vi "main(Test DQMH modules).vi"() -> ()   [LabVIEW 2018, in "Application.lvlib"] (continued)
          }
        }
        n5217 = for {
          tunnel: w11392 -> [w11487] mode=indexing
          tunnel: w11400 -> [w11488]
          tunnel: [w11484] -> w11402 mode=indexing
          n5218 = Unbundle By Name(w11487) -> ("command"=w11486:string, "data"=w11485:variant)
          n5219 = call "App enquece.vi"("command data"=w11485, "command"=w11486, "queue in"=w11488) -> ("error out"=w11484:errorcluster)  [unwired: 7 in, 1 out]
        }
        n5220 = Merge Errors(w11403, w11402) -> (w11401:errorcluster)
      }
      frame "Test DRV 17A" {
        w11492 = 17 ("DUT index(0-59)")
        n5221 = disable-structure shown="LOGGING==TRUE" {
          disable-tunnel: w11497 -> [w11580 _]
          frame condition #0 (active) {
            n5222 = Empty String/Path?(string/path=w11580) -> (empty?=w11582:bool)
            n5223 = Select(t="Quece timeout", s=w11582, f=w11580) -> (s? t:f=w11579:string)
            n5224 = call "string log (SubVI).vi"("state Name"=w11579) -> ()  [unwired: 9 in, 2 out]
          }
          frame condition #1 {
          }
        }
        n5225 = Flush Queue(queue=w11498) -> (queue out=w11499:refnum<queue>)  [unwired: 1 in, 2 out]
        n5226 = Decrement(x=w11492) -> (x-1=w11496:i32)
        n5227 = Index Array(array=w11493, index=w11496) -> (element=w11494:refnum<vi>)
        n5228 = call "FGV DRV stand.vi"() -> ("Sub-Test.DCV"=w11489:bool)  [unwired: 10 in, 1 out]
        n5229 = call "FGV Driver Data.vi"("DUT index(1-60)"=w11492) -> ("DUT SC"=w11490:bool)  [unwired: 7 in, 3 out]
        n5230 = property class="ColBox"(reference=w11494, "Value"=u32 10000536 ("DRV 1")) -> ()  [unwired: 1 in, 2 out]
        n5231 = case shown="False" w11490 {
          tunnel: w11492 -> [w11510 _]
          tunnel: [w11509 w11575] -> w11491
          tunnel: w11489 -> [w11508 _]
          frame False {
            n5232 = case shown="True" w11508 {
              tunnel: w11510 -> [w11517 w11547]
              tunnel: [w11528 w11546] -> w11509
              frame False {
                w11514 = T9 {"command"="", "data"=variant} ("element")
                w11527 = T9 {"command"="", "data"=variant} ("element")
                n5233 = To Variant(anything=T3."mux10_1_channel3" ("mux10_1(x6)_encode")) -> (Variant=w11525:variant)
                n5234 = To Variant(anything=T4."demux1_10_channel3" ("demux1_10(x6)_encode")) -> (Variant=w11521:variant)
                n5235 = To Variant(anything=bool[] [FALSE, FALSE, FALSE, FALSE, TRUE, FALSE]) -> (Variant=w11536:variant)
                n5236 = Bundle By Name(cluster=w11527, "command"="MEAS.AllRelaysOFF") -> (w11535:T9)
                n5237 = Bundle By Name(cluster=w11527, "command"="MEAS.mux10-1", "data"=w11525) -> (w11518:T9)
                n5238 = Bundle By Name(cluster=w11527, "command"="MEAS.demux1-10", "data"=w11521) -> (w11519:T9)
                n5239 = Bundle By Name(cluster=w11527, "command"="MEAS.eMIC", "data"=w11536) -> (w11520:T9)
                n5240 = Build Array(w11535, w11518, w11519, w11520) -> (w11513:T9[])
                n5241 = To Variant(anything=w11517) -> (Variant=w11516:variant)
                n5242 = To Variant(anything=w11517) -> (Variant=w11515:variant)
                n5243 = Bundle By Name(cluster=w11514, "command"="MEAS.requestAC", "data"=w11516) -> (w11533:T9)
                n5244 = Bundle By Name(cluster=w11514, "command"="Apps.WaitForEvent", "data"=w11515) -> (w11529:T9)
                n5245 = Bundle By Name(cluster=w11514, "command"="Apps.UI Update 1") -> (w11530:T9)
                n5246 = Bundle By Name(cluster=w11514, "command"="WaitFor") -> (w11512:T9)
                n5247 = Build Array (concatenate)(w11513, w11512, w11533, w11529, w11530) -> (w11528:T9[])
              }
              frame True {
                w11543 = T9 {"command"="", "data"=variant} ("element")
                w11565 = T9 {"command"="", "data"=variant} ("element")
                n5248 = To Variant(anything=T3."mux10_1_channel3" ("mux10_1(x6)_encode")) -> (Variant=w11572:variant)
                n5249 = To Variant(anything=T2."mux6_1_channel5_3" ("mux6_1(3wires)_encode")) -> (Variant=w11570:variant)
                n5250 = To Variant(anything=T4."demux1_10_channel3" ("demux1_10(x6)_encode")) -> (Variant=w11566:variant)
                n5251 = To Variant(anything=bool[] [FALSE, FALSE, FALSE, FALSE, TRUE, FALSE]) -> (Variant=w11562:variant)
                n5252 = Bundle By Name(cluster=w11565, "command"="MEAS.AllRelaysOFF") -> (w11561:T9)
                n5253 = Bundle By Name(cluster=w11565, "command"="MEAS.mux10-1", "data"=w11572) -> (w11560:T9)
                n5254 = Bundle By Name(cluster=w11565, "command"="MEAS.mux6_1", "data"=w11570) -> (w11559:T9)
                n5255 = Bundle By Name(cluster=w11565, "command"="MEAS.demux1-10", "data"=w11566) -> (w11558:T9)
                n5256 = Bundle By Name(cluster=w11565, "command"="MEAS.eMIC", "data"=w11562) -> (w11557:T9)
                n5257 = Build Array(w11561, w11560, w11559, w11558, w11557) -> (w11542:T9[])
                n5258 = To Variant(anything=w11547) -> (Variant=w11545:variant)
                n5259 = To Variant(anything=w11547) -> (Variant=w11544:variant)
                n5260 = Bundle By Name(cluster=w11543, "command"="WaitFor") -> (w11541:T9)
                n5261 = Bundle By Name(cluster=w11543, "command"="MEAS.DMM dual read") -> (w11554:T9)
                n5262 = Bundle By Name(cluster=w11543, "command"="MEAS.requestAC", "data"=w11545) -> (w11553:T9)
                n5263 = Bundle By Name(cluster=w11543, "command"="Apps.WaitForEvent", "data"=w11544) -> (w11548:T9)
                n5264 = Bundle By Name(cluster=w11543, "command"="Apps.UI Update 1") -> (w11549:T9)
                n5265 = Build Array (concatenate)(w11542, w11541, w11554, w11553, w11548, w11549) -> (w11546:T9[])
              }
            }
          }
          frame True {
            n5266 = Bundle By Name(cluster=T9 {"command"="", "data"=variant} ("element"), "command"="Apps.UI Update 1") -> (w11576:T9)
            n5267 = Build Array(w11576) -> (w11575:T9[])
          }
        }
        n5268 = for {
          tunnel: w11491 -> [w11586] mode=indexing
          tunnel: w11499 -> [w11587]
          tunnel: [w11583] -> w11501 mode=indexing
          n5269 = Unbundle By Name(w11586) -> ("command"=w11585:string, "data"=w11584:variant)
          n5270 = call "App enquece.vi"("command data"=w11584, "command"=w11585, "queue in"=w11587) -> ("error out"=w11583:errorcluster)  [unwired: 7 in, 1 out]
        }
        n5271 = Merge Errors(w11502, w11501) -> (w11500:errorcluster)
      }
      frame "Test DRV 18A" {
        w11591 = 18 ("DUT index(0-59)")
        n5272 = disable-structure shown="LOGGING==TRUE" {
          disable-tunnel: w11596 -> [w11679 _]
          frame condition #0 (active) {
            n5273 = Empty String/Path?(string/path=w11679) -> (empty?=w11681:bool)
            n5274 = Select(t="Quece timeout", s=w11681, f=w11679) -> (s? t:f=w11678:string)
            n5275 = call "string log (SubVI).vi"("state Name"=w11678) -> ()  [unwired: 9 in, 2 out]
          }
          frame condition #1 {
          }
        }
        n5276 = Flush Queue(queue=w11597) -> (queue out=w11598:refnum<queue>)  [unwired: 1 in, 2 out]
        n5277 = Decrement(x=w11591) -> (x-1=w11595:i32)
        n5278 = Index Array(array=w11592, index=w11595) -> (element=w11593:refnum<vi>)
        n5279 = call "FGV DRV stand.vi"() -> ("Sub-Test.DCV"=w11588:bool)  [unwired: 10 in, 1 out]
        n5280 = call "FGV Driver Data.vi"("DUT index(1-60)"=w11591) -> ("DUT SC"=w11589:bool)  [unwired: 7 in, 3 out]
        n5281 = property class="ColBox"(reference=w11593, "Value"=u32 10000536 ("DRV 1")) -> ()  [unwired: 1 in, 2 out]
        n5282 = case shown="False" w11589 {
          tunnel: w11591 -> [w11609 _]
          tunnel: [w11608 w11674] -> w11590
          tunnel: w11588 -> [w11607 _]
          frame False {
            n5283 = case shown="False" w11607 {
              tunnel: w11609 -> [w11616 w11646]
              tunnel: [w11627 w11645] -> w11608
              frame False {
                w11613 = T9 {"command"="", "data"=variant} ("element")
                w11626 = T9 {"command"="", "data"=variant} ("element")
                n5284 = To Variant(anything=T3."mux10_1_channel3" ("mux10_1(x6)_encode")) -> (Variant=w11624:variant)
                n5285 = To Variant(anything=T4."demux1_10_channel3" ("demux1_10(x6)_encode")) -> (Variant=w11620:variant)
                n5286 = To Variant(anything=bool[] [FALSE, FALSE, FALSE, FALSE, FALSE, TRUE]) -> (Variant=w11635:variant)
                n5287 = Bundle By Name(cluster=w11626, "command"="MEAS.AllRelaysOFF") -> (w11634:T9)
                n5288 = Bundle By Name(cluster=w11626, "command"="MEAS.mux10-1", "data"=w11624) -> (w11617:T9)
                n5289 = Bundle By Name(cluster=w11626, "command"="MEAS.demux1-10", "data"=w11620) -> (w11618:T9)
                n5290 = Bundle By Name(cluster=w11626, "command"="MEAS.eMIC", "data"=w11635) -> (w11619:T9)
                n5291 = Build Array(w11634, w11617, w11618, w11619) -> (w11612:T9[])
                n5292 = To Variant(anything=w11616) -> (Variant=w11615:variant)
                n5293 = To Variant(anything=w11616) -> (Variant=w11614:variant)
                n5294 = Bundle By Name(cluster=w11613, "command"="MEAS.requestAC", "data"=w11615) -> (w11632:T9)
                n5295 = Bundle By Name(cluster=w11613, "command"="Apps.WaitForEvent", "data"=w11614) -> (w11628:T9)
                n5296 = Bundle By Name(cluster=w11613, "command"="Apps.UI Update 1") -> (w11629:T9)
                n5297 = Bundle By Name(cluster=w11613, "command"="WaitFor") -> (w11611:T9)
                n5298 = Build Array (concatenate)(w11612, w11611, w11632, w11628, w11629) -> (w11627:T9[])
              }
              frame True {
                w11642 = T9 {"command"="", "data"=variant} ("element")
                w11664 = T9 {"command"="", "data"=variant} ("element")
                n5299 = To Variant(anything=T3."mux10_1_channel3" ("mux10_1(x6)_encode")) -> (Variant=w11671:variant)
                n5300 = To Variant(anything=T2."mux6_1_channel6_3" ("mux6_1(3wires)_encode")) -> (Variant=w11669:variant)
                n5301 = To Variant(anything=T4."demux1_10_channel3" ("demux1_10(x6)_encode")) -> (Variant=w11665:variant)
                n5302 = To Variant(anything=bool[] [FALSE, FALSE, FALSE, FALSE, FALSE, TRUE]) -> (Variant=w11661:variant)
                n5303 = Bundle By Name(cluster=w11664, "command"="MEAS.AllRelaysOFF") -> (w11660:T9)
                n5304 = Bundle By Name(cluster=w11664, "command"="MEAS.mux10-1", "data"=w11671) -> (w11659:T9)
                n5305 = Bundle By Name(cluster=w11664, "command"="MEAS.mux6_1", "data"=w11669) -> (w11658:T9)
                n5306 = Bundle By Name(cluster=w11664, "command"="MEAS.demux1-10", "data"=w11665) -> (w11657:T9)
                n5307 = Bundle By Name(cluster=w11664, "command"="MEAS.eMIC", "data"=w11661) -> (w11656:T9)
                n5308 = Build Array(w11660, w11659, w11658, w11657, w11656) -> (w11641:T9[])
                n5309 = To Variant(anything=w11646) -> (Variant=w11644:variant)
                n5310 = To Variant(anything=w11646) -> (Variant=w11643:variant)
                n5311 = Bundle By Name(cluster=w11642, "command"="WaitFor") -> (w11640:T9)
                n5312 = Bundle By Name(cluster=w11642, "command"="MEAS.DMM dual read") -> (w11653:T9)
                n5313 = Bundle By Name(cluster=w11642, "command"="MEAS.requestAC", "data"=w11644) -> (w11652:T9)
                n5314 = Bundle By Name(cluster=w11642, "command"="Apps.WaitForEvent", "data"=w11643) -> (w11647:T9)
                n5315 = Bundle By Name(cluster=w11642, "command"="Apps.UI Update 1") -> (w11648:T9)
                n5316 = Build Array (concatenate)(w11641, w11640, w11653, w11652, w11647, w11648) -> (w11645:T9[])
              }
            }
          }
          frame True {
            n5317 = Bundle By Name(cluster=T9 {"command"="", "data"=variant} ("element"), "command"="Apps.UI Update 1") -> (w11675:T9)
            n5318 = Build Array(w11675) -> (w11674:T9[])
          }
        }
        n5319 = for {
          tunnel: w11590 -> [w11685] mode=indexing
          tunnel: w11598 -> [w11686]
          tunnel: [w11682] -> w11600 mode=indexing
          n5320 = Unbundle By Name(w11685) -> ("command"=w11684:string, "data"=w11683:variant)
          n5321 = call "App enquece.vi"("command data"=w11683, "command"=w11684, "queue in"=w11686) -> ("error out"=w11682:errorcluster)  [unwired: 7 in, 1 out]
        }
        n5322 = Merge Errors(w11601, w11600) -> (w11599:errorcluster)
      }
      frame "Test DRV 19A" {
        w11690 = 19 ("DUT index(0-59)")
        n5323 = disable-structure shown="LOGGING==TRUE" {
          disable-tunnel: w11695 -> [w11778 _]
          frame condition #0 (active) {
            n5324 = Empty String/Path?(string/path=w11778) -> (empty?=w11780:bool)
            n5325 = Select(t="Quece timeout", s=w11780, f=w11778) -> (s? t:f=w11777:string)
            n5326 = call "string log (SubVI).vi"("state Name"=w11777) -> ()  [unwired: 9 in, 2 out]
          }
          frame condition #1 {
          }
        }
        n5327 = Flush Queue(queue=w11696) -> (queue out=w11697:refnum<queue>)  [unwired: 1 in, 2 out]
        n5328 = Decrement(x=w11690) -> (x-1=w11694:i32)
        n5329 = Index Array(array=w11691, index=w11694) -> (element=w11692:refnum<vi>)
        n5330 = call "FGV DRV stand.vi"() -> ("Sub-Test.DCV"=w11687:bool)  [unwired: 10 in, 1 out]
        n5331 = call "FGV Driver Data.vi"("DUT index(1-60)"=w11690) -> ("DUT SC"=w11688:bool)  [unwired: 7 in, 3 out]
        n5332 = property class="ColBox"(reference=w11692, "Value"=u32 10000536 ("DRV 1")) -> ()  [unwired: 1 in, 2 out]
        n5333 = case shown="False" w11688 {
          tunnel: w11690 -> [w11708 _]
          tunnel: [w11707 w11773] -> w11689
          tunnel: w11687 -> [w11706 _]
          frame False {
            n5334 = case shown="True" w11706 {
              tunnel: w11708 -> [w11715 w11745]
              tunnel: [w11726 w11744] -> w11707
              frame False {
                w11712 = T9 {"command"="", "data"=variant} ("element")
                w11725 = T9 {"command"="", "data"=variant} ("element")
                n5335 = To Variant(anything=T3."mux10_1_channel4" ("mux10_1(x6)_encode")) -> (Variant=w11723:variant)
                n5336 = To Variant(anything=T4."demux1_10_channel4" ("demux1_10(x6)_encode")) -> (Variant=w11719:variant)
                n5337 = To Variant(anything=bool[] [TRUE, FALSE, FALSE, FALSE, FALSE, FALSE]) -> (Variant=w11734:variant)
                n5338 = Bundle By Name(cluster=w11725, "command"="MEAS.AllRelaysOFF") -> (w11733:T9)
                n5339 = Bundle By Name(cluster=w11725, "command"="MEAS.mux10-1", "data"=w11723) -> (w11716:T9)
                n5340 = Bundle By Name(cluster=w11725, "command"="MEAS.demux1-10", "data"=w11719) -> (w11717:T9)
                n5341 = Bundle By Name(cluster=w11725, "command"="MEAS.eMIC", "data"=w11734) -> (w11718:T9)
                n5342 = Build Array(w11733, w11716, w11717, w11718) -> (w11711:T9[])
                n5343 = To Variant(anything=w11715) -> (Variant=w11714:variant)
                n5344 = To Variant(anything=w11715) -> (Variant=w11713:variant)
                n5345 = Bundle By Name(cluster=w11712, "command"="MEAS.requestAC", "data"=w11714) -> (w11731:T9)
                n5346 = Bundle By Name(cluster=w11712, "command"="Apps.WaitForEvent", "data"=w11713) -> (w11727:T9)
                n5347 = Bundle By Name(cluster=w11712, "command"="Apps.UI Update 1") -> (w11728:T9)
                n5348 = Bundle By Name(cluster=w11712, "command"="WaitFor") -> (w11710:T9)
                n5349 = Build Array (concatenate)(w11711, w11710, w11731, w11727, w11728) -> (w11726:T9[])
              }
              frame True {
                w11741 = T9 {"command"="", "data"=variant} ("element")
                w11763 = T9 {"command"="", "data"=variant} ("element")
                n5350 = To Variant(anything=T3."mux10_1_channel4" ("mux10_1(x6)_encode")) -> (Variant=w11770:variant)
                n5351 = To Variant(anything=T2."mux6_1_channel1_3" ("mux6_1(3wires)_encode")) -> (Variant=w11768:variant)
                n5352 = To Variant(anything=T4."demux1_10_channel4" ("demux1_10(x6)_encode")) -> (Variant=w11764:variant)
                n5353 = To Variant(anything=bool[] [TRUE, FALSE, FALSE, FALSE, FALSE, FALSE]) -> (Variant=w11760:variant)
                n5354 = Bundle By Name(cluster=w11763, "command"="MEAS.AllRelaysOFF") -> (w11759:T9)
                n5355 = Bundle By Name(cluster=w11763, "command"="MEAS.mux10-1", "data"=w11770) -> (w11758:T9)
                n5356 = Bundle By Name(cluster=w11763, "command"="MEAS.mux6_1", "data"=w11768) -> (w11757:T9)
                n5357 = Bundle By Name(cluster=w11763, "command"="MEAS.demux1-10", "data"=w11764) -> (w11756:T9)
                n5358 = Bundle By Name(cluster=w11763, "command"="MEAS.eMIC", "data"=w11760) -> (w11755:T9)
                n5359 = Build Array(w11759, w11758, w11757, w11756, w11755) -> (w11740:T9[])
                n5360 = To Variant(anything=w11745) -> (Variant=w11743:variant)
                n5361 = To Variant(anything=w11745) -> (Variant=w11742:variant)
                n5362 = Bundle By Name(cluster=w11741, "command"="WaitFor") -> (w11739:T9)
                n5363 = Bundle By Name(cluster=w11741, "command"="MEAS.DMM dual read") -> (w11752:T9)
                n5364 = Bundle By Name(cluster=w11741, "command"="MEAS.requestAC", "data"=w11743) -> (w11751:T9)
                n5365 = Bundle By Name(cluster=w11741, "command"="Apps.WaitForEvent", "data"=w11742) -> (w11746:T9)
                n5366 = Bundle By Name(cluster=w11741, "command"="Apps.UI Update 1") -> (w11747:T9)
                n5367 = Build Array (concatenate)(w11740, w11739, w11752, w11751, w11746, w11747) -> (w11744:T9[])
              }
            }
          }
          frame True {
            n5368 = Bundle By Name(cluster=T9 {"command"="", "data"=variant} ("element"), "command"="Apps.UI Update 1") -> (w11774:T9)
            n5369 = Build Array(w11774) -> (w11773:T9[])
          }
        }
        n5370 = for {
          tunnel: w11689 -> [w11784] mode=indexing
          tunnel: w11697 -> [w11785]
          tunnel: [w11781] -> w11699 mode=indexing
          n5371 = Unbundle By Name(w11784) -> ("command"=w11783:string, "data"=w11782:variant)
          n5372 = call "App enquece.vi"("command data"=w11782, "command"=w11783, "queue in"=w11785) -> ("error out"=w11781:errorcluster)  [unwired: 7 in, 1 out]
        }
        n5373 = Merge Errors(w11700, w11699) -> (w11698:errorcluster)
      }
      frame "Test DRV 20A" {
        w11789 = 20 ("DUT index(0-59)")
        n5374 = disable-structure shown="LOGGING==TRUE" {
          disable-tunnel: w11794 -> [w11877 _]
          frame condition #0 (active) {
            n5375 = Empty String/Path?(string/path=w11877) -> (empty?=w11879:bool)
            n5376 = Select(t="Quece timeout", s=w11879, f=w11877) -> (s? t:f=w11876:string)
            n5377 = call "string log (SubVI).vi"("state Name"=w11876) -> ()  [unwired: 9 in, 2 out]
          }
          frame condition #1 {
          }
        }
        n5378 = Flush Queue(queue=w11795) -> (queue out=w11796:refnum<queue>)  [unwired: 1 in, 2 out]
        n5379 = Decrement(x=w11789) -> (x-1=w11793:i32)
        n5380 = Index Array(array=w11790, index=w11793) -> (element=w11791:refnum<vi>)
        n5381 = call "FGV DRV stand.vi"() -> ("Sub-Test.DCV"=w11786:bool)  [unwired: 10 in, 1 out]
        n5382 = call "FGV Driver Data.vi"("DUT index(1-60)"=w11789) -> ("DUT SC"=w11787:bool)  [unwired: 7 in, 3 out]
        n5383 = property class="ColBox"(reference=w11791, "Value"=u32 10000536 ("DRV 1")) -> ()  [unwired: 1 in, 2 out]
        n5384 = case shown="False" w11787 {
          tunnel: w11789 -> [w11807 _]
          tunnel: [w11806 w11872] -> w11788
          tunnel: w11786 -> [w11805 _]
          frame False {
            n5385 = case shown="False" w11805 {
              tunnel: w11807 -> [w11814 w11844]
              tunnel: [w11825 w11843] -> w11806
              frame False {
                w11811 = T9 {"command"="", "data"=variant} ("element")
                w11824 = T9 {"command"="", "data"=variant} ("element")
                n5386 = To Variant(anything=T3."mux10_1_channel4" ("mux10_1(x6)_encode")) -> (Variant=w11822:variant)
                n5387 = To Variant(anything=T4."demux1_10_channel4" ("demux1_10(x6)_encode")) -> (Variant=w11818:variant)
                n5388 = To Variant(anything=bool[] [FALSE, TRUE, FALSE, FALSE, FALSE, FALSE]) -> (Variant=w11833:variant)
                n5389 = Bundle By Name(cluster=w11824, "command"="MEAS.AllRelaysOFF") -> (w11832:T9)
                n5390 = Bundle By Name(cluster=w11824, "command"="MEAS.mux10-1", "data"=w11822) -> (w11815:T9)
                n5391 = Bundle By Name(cluster=w11824, "command"="MEAS.demux1-10", "data"=w11818) -> (w11816:T9)
                n5392 = Bundle By Name(cluster=w11824, "command"="MEAS.eMIC", "data"=w11833) -> (w11817:T9)
                n5393 = Build Array(w11832, w11815, w11816, w11817) -> (w11810:T9[])
                n5394 = To Variant(anything=w11814) -> (Variant=w11813:variant)
                n5395 = To Variant(anything=w11814) -> (Variant=w11812:variant)
                n5396 = Bundle By Name(cluster=w11811, "command"="MEAS.requestAC", "data"=w11813) -> (w11830:T9)
                n5397 = Bundle By Name(cluster=w11811, "command"="Apps.WaitForEvent", "data"=w11812) -> (w11826:T9)
                n5398 = Bundle By Name(cluster=w11811, "command"="Apps.UI Update 1") -> (w11827:T9)
                n5399 = Bundle By Name(cluster=w11811, "command"="WaitFor") -> (w11809:T9)
                n5400 = Build Array (concatenate)(w11810, w11809, w11830, w11826, w11827) -> (w11825:T9[])
              }
              frame True {
                w11840 = T9 {"command"="", "data"=variant} ("element")
                w11862 = T9 {"command"="", "data"=variant} ("element")
                n5401 = To Variant(anything=T3."mux10_1_channel4" ("mux10_1(x6)_encode")) -> (Variant=w11869:variant)
                n5402 = To Variant(anything=T2."mux6_1_channel2_3" ("mux6_1(3wires)_encode")) -> (Variant=w11867:variant)
                n5403 = To Variant(anything=T4."demux1_10_channel4" ("demux1_10(x6)_encode")) -> (Variant=w11863:variant)
                n5404 = To Variant(anything=bool[] [FALSE, TRUE, FALSE, FALSE, FALSE, FALSE]) -> (Variant=w11859:variant)
                n5405 = Bundle By Name(cluster=w11862, "command"="MEAS.AllRelaysOFF") -> (w11858:T9)
                n5406 = Bundle By Name(cluster=w11862, "command"="MEAS.mux10-1", "data"=w11869) -> (w11857:T9)
                n5407 = Bundle By Name(cluster=w11862, "command"="MEAS.mux6_1", "data"=w11867) -> (w11856:T9)
                n5408 = Bundle By Name(cluster=w11862, "command"="MEAS.demux1-10", "data"=w11863) -> (w11855:T9)
                n5409 = Bundle By Name(cluster=w11862, "command"="MEAS.eMIC", "data"=w11859) -> (w11854:T9)
                n5410 = Build Array(w11858, w11857, w11856, w11855, w11854) -> (w11839:T9[])
                n5411 = To Variant(anything=w11844) -> (Variant=w11842:variant)
                n5412 = To Variant(anything=w11844) -> (Variant=w11841:variant)
                n5413 = Bundle By Name(cluster=w11840, "command"="WaitFor") -> (w11838:T9)
                n5414 = Bundle By Name(cluster=w11840, "command"="MEAS.DMM dual read") -> (w11851:T9)
                n5415 = Bundle By Name(cluster=w11840, "command"="MEAS.requestAC", "data"=w11842) -> (w11850:T9)
                n5416 = Bundle By Name(cluster=w11840, "command"="Apps.WaitForEvent", "data"=w11841) -> (w11845:T9)
                n5417 = Bundle By Name(cluster=w11840, "command"="Apps.UI Update 1") -> (w11846:T9)
                n5418 = Build Array (concatenate)(w11839, w11838, w11851, w11850, w11845, w11846) -> (w11843:T9[])
              }
            }
          }
          frame True {
            n5419 = Bundle By Name(cluster=T9 {"command"="", "data"=variant} ("element"), "command"="Apps.UI Update 1") -> (w11873:T9)
            n5420 = Build Array(w11873) -> (w11872:T9[])
          }
        }
        n5421 = for {
          tunnel: w11788 -> [w11883] mode=indexing
          tunnel: w11796 -> [w11884]
          tunnel: [w11880] -> w11798 mode=indexing
          n5422 = Unbundle By Name(w11883) -> ("command"=w11882:string, "data"=w11881:variant)
          n5423 = call "App enquece.vi"("command data"=w11881, "command"=w11882, "queue in"=w11884) -> ("error out"=w11880:errorcluster)  [unwired: 7 in, 1 out]
        }
        n5424 = Merge Errors(w11799, w11798) -> (w11797:errorcluster)
      }
      frame "Test DRV 21A" {
        w11888 = 21 ("DUT index(0-59)")
        n5425 = disable-structure shown="LOGGING==TRUE" {
          disable-tunnel: w11893 -> [w11976 _]
          frame condition #0 (active) {
            n5426 = Empty String/Path?(string/path=w11976) -> (empty?=w11978:bool)
            n5427 = Select(t="Quece timeout", s=w11978, f=w11976) -> (s? t:f=w11975:string)
            n5428 = call "string log (SubVI).vi"("state Name"=w11975) -> ()  [unwired: 9 in, 2 out]
          }
          frame condition #1 {
          }
        }
        n5429 = Flush Queue(queue=w11894) -> (queue out=w11895:refnum<queue>)  [unwired: 1 in, 2 out]
        n5430 = Decrement(x=w11888) -> (x-1=w11892:i32)
        n5431 = Index Array(array=w11889, index=w11892) -> (element=w11890:refnum<vi>)
        n5432 = call "FGV DRV stand.vi"() -> ("Sub-Test.DCV"=w11885:bool)  [unwired: 10 in, 1 out]
        n5433 = call "FGV Driver Data.vi"("DUT index(1-60)"=w11888) -> ("DUT SC"=w11886:bool)  [unwired: 7 in, 3 out]
        n5434 = property class="ColBox"(reference=w11890, "Value"=u32 10000536 ("DRV 1")) -> ()  [unwired: 1 in, 2 out]
        n5435 = case shown="False" w11886 {
          tunnel: w11888 -> [w11906 _]
          tunnel: [w11905 w11971] -> w11887
          tunnel: w11885 -> [w11904 _]
          frame False {
            n5436 = case shown="True" w11904 {
              tunnel: w11906 -> [w11913 w11943]
              tunnel: [w11924 w11942] -> w11905
              frame False {
                w11910 = T9 {"command"="", "data"=variant} ("element")
                w11923 = T9 {"command"="", "data"=variant} ("element")
                n5437 = To Variant(anything=T3."mux10_1_channel4" ("mux10_1(x6)_encode")) -> (Variant=w11921:variant)
                n5438 = To Variant(anything=T4."demux1_10_channel4" ("demux1_10(x6)_encode")) -> (Variant=w11917:variant)
                n5439 = To Variant(anything=bool[] [FALSE, FALSE, TRUE, FALSE, FALSE, FALSE]) -> (Variant=w11932:variant)
                n5440 = Bundle By Name(cluster=w11923, "command"="MEAS.AllRelaysOFF") -> (w11931:T9)
                n5441 = Bundle By Name(cluster=w11923, "command"="MEAS.mux10-1", "data"=w11921) -> (w11914:T9)
                n5442 = Bundle By Name(cluster=w11923, "command"="MEAS.demux1-10", "data"=w11917) -> (w11915:T9)
                n5443 = Bundle By Name(cluster=w11923, "command"="MEAS.eMIC", "data"=w11932) -> (w11916:T9)
                n5444 = Build Array(w11931, w11914, w11915, w11916) -> (w11909:T9[])
                n5445 = To Variant(anything=w11913) -> (Variant=w11912:variant)
                n5446 = To Variant(anything=w11913) -> (Variant=w11911:variant)
                n5447 = Bundle By Name(cluster=w11910, "command"="MEAS.requestAC", "data"=w11912) -> (w11929:T9)
                n5448 = Bundle By Name(cluster=w11910, "command"="Apps.WaitForEvent", "data"=w11911) -> (w11925:T9)
                n5449 = Bundle By Name(cluster=w11910, "command"="Apps.UI Update 1") -> (w11926:T9)
                n5450 = Bundle By Name(cluster=w11910, "command"="WaitFor") -> (w11908:T9)
                n5451 = Build Array (concatenate)(w11909, w11908, w11929, w11925, w11926) -> (w11924:T9[])
              }
              frame True {
                w11939 = T9 {"command"="", "data"=variant} ("element")
                w11961 = T9 {"command"="", "data"=variant} ("element")
                n5452 = To Variant(anything=T3."mux10_1_channel4" ("mux10_1(x6)_encode")) -> (Variant=w11968:variant)
                n5453 = To Variant(anything=T2."mux6_1_channel3_3" ("mux6_1(3wires)_encode")) -> (Variant=w11966:variant)
                n5454 = To Variant(anything=T4."demux1_10_channel4" ("demux1_10(x6)_encode")) -> (Variant=w11962:variant)
                n5455 = To Variant(anything=bool[] [FALSE, FALSE, TRUE, FALSE, FALSE, FALSE]) -> (Variant=w11958:variant)
                n5456 = Bundle By Name(cluster=w11961, "command"="MEAS.AllRelaysOFF") -> (w11957:T9)
                n5457 = Bundle By Name(cluster=w11961, "command"="MEAS.mux10-1", "data"=w11968) -> (w11956:T9)
                n5458 = Bundle By Name(cluster=w11961, "command"="MEAS.mux6_1", "data"=w11966) -> (w11955:T9)
                n5459 = Bundle By Name(cluster=w11961, "command"="MEAS.demux1-10", "data"=w11962) -> (w11954:T9)
                n5460 = Bundle By Name(cluster=w11961, "command"="MEAS.eMIC", "data"=w11958) -> (w11953:T9)
                n5461 = Build Array(w11957, w11956, w11955, w11954, w11953) -> (w11938:T9[])
                n5462 = To Variant(anything=w11943) -> (Variant=w11941:variant)
                n5463 = To Variant(anything=w11943) -> (Variant=w11940:variant)
                n5464 = Bundle By Name(cluster=w11939, "command"="WaitFor") -> (w11937:T9)
                n5465 = Bundle By Name(cluster=w11939, "command"="MEAS.DMM dual read") -> (w11950:T9)
                n5466 = Bundle By Name(cluster=w11939, "command"="MEAS.requestAC", "data"=w11941) -> (w11949:T9)
                n5467 = Bundle By Name(cluster=w11939, "command"="Apps.WaitForEvent", "data"=w11940) -> (w11944:T9)
                n5468 = Bundle By Name(cluster=w11939, "command"="Apps.UI Update 1") -> (w11945:T9)
                n5469 = Build Array (concatenate)(w11938, w11937, w11950, w11949, w11944, w11945) -> (w11942:T9[])
              }
            }
          }
          frame True {
            n5470 = Bundle By Name(cluster=T9 {"command"="", "data"=variant} ("element"), "command"="Apps.UI Update 1") -> (w11972:T9)
            n5471 = Build Array(w11972) -> (w11971:T9[])
          }
        }
        n5472 = for {
          tunnel: w11887 -> [w11982] mode=indexing
          tunnel: w11895 -> [w11983]
          tunnel: [w11979] -> w11897 mode=indexing
          n5473 = Unbundle By Name(w11982) -> ("command"=w11981:string, "data"=w11980:variant)
          n5474 = call "App enquece.vi"("command data"=w11980, "command"=w11981, "queue in"=w11983) -> ("error out"=w11979:errorcluster)  [unwired: 7 in, 1 out]
        }
        n5475 = Merge Errors(w11898, w11897) -> (w11896:errorcluster)
      }
      frame "Test DRV 22A" {
        w11987 = 22 ("DUT index(0-59)")
        n5476 = disable-structure shown="LOGGING==TRUE" {
          disable-tunnel: w11992 -> [w12075 _]
          frame condition #0 (active) {
            n5477 = Empty String/Path?(string/path=w12075) -> (empty?=w12077:bool)
            n5478 = Select(t="Quece timeout", s=w12077, f=w12075) -> (s? t:f=w12074:string)
            n5479 = call "string log (SubVI).vi"("state Name"=w12074) -> ()  [unwired: 9 in, 2 out]
          }
          frame condition #1 {
          }
        }
        n5480 = Flush Queue(queue=w11993) -> (queue out=w11994:refnum<queue>)  [unwired: 1 in, 2 out]
        n5481 = Decrement(x=w11987) -> (x-1=w11991:i32)
        n5482 = Index Array(array=w11988, index=w11991) -> (element=w11989:refnum<vi>)
        n5483 = call "FGV DRV stand.vi"() -> ("Sub-Test.DCV"=w11984:bool)  [unwired: 10 in, 1 out]
        n5484 = call "FGV Driver Data.vi"("DUT index(1-60)"=w11987) -> ("DUT SC"=w11985:bool)  [unwired: 7 in, 3 out]
        n5485 = property class="ColBox"(reference=w11989, "Value"=u32 10000536 ("DRV 1")) -> ()  [unwired: 1 in, 2 out]
        n5486 = case shown="False" w11985 {
          tunnel: w11987 -> [w12005 _]
          tunnel: [w12004 w12070] -> w11986
          tunnel: w11984 -> [w12003 _]
          frame False {
            n5487 = case shown="False" w12003 {
              tunnel: w12005 -> [w12012 w12042]
              tunnel: [w12023 w12041] -> w12004
              frame False {
                w12009 = T9 {"command"="", "data"=variant} ("element")
                w12022 = T9 {"command"="", "data"=variant} ("element")
                n5488 = To Variant(anything=T3."mux10_1_channel4" ("mux10_1(x6)_encode")) -> (Variant=w12020:variant)
                n5489 = To Variant(anything=T4."demux1_10_channel4" ("demux1_10(x6)_encode")) -> (Variant=w12016:variant)
                n5490 = To Variant(anything=bool[] [FALSE, FALSE, FALSE, TRUE, FALSE, FALSE]) -> (Variant=w12031:variant)
                n5491 = Bundle By Name(cluster=w12022, "command"="MEAS.AllRelaysOFF") -> (w12030:T9)
                n5492 = Bundle By Name(cluster=w12022, "command"="MEAS.mux10-1", "data"=w12020) -> (w12013:T9)
                n5493 = Bundle By Name(cluster=w12022, "command"="MEAS.demux1-10", "data"=w12016) -> (w12014:T9)
                n5494 = Bundle By Name(cluster=w12022, "command"="MEAS.eMIC", "data"=w12031) -> (w12015:T9)
                n5495 = Build Array(w12030, w12013, w12014, w12015) -> (w12008:T9[])
                n5496 = To Variant(anything=w12012) -> (Variant=w12011:variant)
                n5497 = To Variant(anything=w12012) -> (Variant=w12010:variant)
                n5498 = Bundle By Name(cluster=w12009, "command"="MEAS.requestAC", "data"=w12011) -> (w12028:T9)
                n5499 = Bundle By Name(cluster=w12009, "command"="Apps.WaitForEvent", "data"=w12010) -> (w12024:T9)
                n5500 = Bundle By Name(cluster=w12009, "command"="Apps.UI Update 1") -> (w12025:T9)
                n5501 = Bundle By Name(cluster=w12009, "command"="WaitFor") -> (w12007:T9)
                n5502 = Build Array (concatenate)(w12008, w12007, w12028, w12024, w12025) -> (w12023:T9[])
              }
              frame True {
                w12038 = T9 {"command"="", "data"=variant} ("element")
                w12060 = T9 {"command"="", "data"=variant} ("element")
                n5503 = To Variant(anything=T3."mux10_1_channel4" ("mux10_1(x6)_encode")) -> (Variant=w12067:variant)
                n5504 = To Variant(anything=T2."mux6_1_channel4_3" ("mux6_1(3wires)_encode")) -> (Variant=w12065:variant)
                n5505 = To Variant(anything=T4."demux1_10_channel4" ("demux1_10(x6)_encode")) -> (Variant=w12061:variant)
                n5506 = To Variant(anything=bool[] [FALSE, FALSE, FALSE, TRUE, FALSE, FALSE]) -> (Variant=w12057:variant)
                n5507 = Bundle By Name(cluster=w12060, "command"="MEAS.AllRelaysOFF") -> (w12056:T9)
                n5508 = Bundle By Name(cluster=w12060, "command"="MEAS.mux10-1", "data"=w12067) -> (w12055:T9)
                n5509 = Bundle By Name(cluster=w12060, "command"="MEAS.mux6_1", "data"=w12065) -> (w12054:T9)
                n5510 = Bundle By Name(cluster=w12060, "command"="MEAS.demux1-10", "data"=w12061) -> (w12053:T9)
                n5511 = Bundle By Name(cluster=w12060, "command"="MEAS.eMIC", "data"=w12057) -> (w12052:T9)
                n5512 = Build Array(w12056, w12055, w12054, w12053, w12052) -> (w12037:T9[])
                n5513 = To Variant(anything=w12042) -> (Variant=w12040:variant)
                n5514 = To Variant(anything=w12042) -> (Variant=w12039:variant)
                n5515 = Bundle By Name(cluster=w12038, "command"="WaitFor") -> (w12036:T9)
                n5516 = Bundle By Name(cluster=w12038, "command"="MEAS.DMM dual read") -> (w12049:T9)
                n5517 = Bundle By Name(cluster=w12038, "command"="MEAS.requestAC", "data"=w12040) -> (w12048:T9)
                n5518 = Bundle By Name(cluster=w12038, "command"="Apps.WaitForEvent", "data"=w12039) -> (w12043:T9)
                n5519 = Bundle By Name(cluster=w12038, "command"="Apps.UI Update 1") -> (w12044:T9)
                n5520 = Build Array (concatenate)(w12037, w12036, w12049, w12048, w12043, w12044) -> (w12041:T9[])
              }
            }
          }
          frame True {
            n5521 = Bundle By Name(cluster=T9 {"command"="", "data"=variant} ("element"), "command"="Apps.UI Update 1") -> (w12071:T9)
            n5522 = Build Array(w12071) -> (w12070:T9[])
          }
        }
        n5523 = for {
          tunnel: w11986 -> [w12081] mode=indexing
          tunnel: w11994 -> [w12082]
          tunnel: [w12078] -> w11996 mode=indexing
          n5524 = Unbundle By Name(w12081) -> ("command"=w12080:string, "data"=w12079:variant)
          n5525 = call "App enquece.vi"("command data"=w12079, "command"=w12080, "queue in"=w12082) -> ("error out"=w12078:errorcluster)  [unwired: 7 in, 1 out]
        }
        n5526 = Merge Errors(w11997, w11996) -> (w11995:errorcluster)
      }
      frame "Test DRV 23A" {
        w12086 = 23 ("DUT index(0-59)")
        n5527 = disable-structure shown="LOGGING==TRUE" {
          disable-tunnel: w12091 -> [w12174 _]
          frame condition #0 (active) {
            n5528 = Empty String/Path?(string/path=w12174) -> (empty?=w12176:bool)
            n5529 = Select(t="Quece timeout", s=w12176, f=w12174) -> (s? t:f=w12173:string)
            n5530 = call "string log (SubVI).vi"("state Name"=w12173) -> ()  [unwired: 9 in, 2 out]
          }
          frame condition #1 {
          }
        }
        n5531 = Flush Queue(queue=w12092) -> (queue out=w12093:refnum<queue>)  [unwired: 1 in, 2 out]
        n5532 = Decrement(x=w12086) -> (x-1=w12090:i32)
        n5533 = Index Array(array=w12087, index=w12090) -> (element=w12088:refnum<vi>)
        n5534 = call "FGV DRV stand.vi"() -> ("Sub-Test.DCV"=w12083:bool)  [unwired: 10 in, 1 out]
        n5535 = call "FGV Driver Data.vi"("DUT index(1-60)"=w12086) -> ("DUT SC"=w12084:bool)  [unwired: 7 in, 3 out]
        n5536 = property class="ColBox"(reference=w12088, "Value"=u32 10000536 ("DRV 1")) -> ()  [unwired: 1 in, 2 out]
        n5537 = case shown="False" w12084 {
          tunnel: w12086 -> [w12104 _]
          tunnel: [w12103 w12169] -> w12085
          tunnel: w12083 -> [w12102 _]
          frame False {
            n5538 = case shown="True" w12102 {
              tunnel: w12104 -> [w12111 w12141]
              tunnel: [w12122 w12140] -> w12103
              frame False {
                w12108 = T9 {"command"="", "data"=variant} ("element")
                w12121 = T9 {"command"="", "data"=variant} ("element")
                n5539 = To Variant(anything=T3."mux10_1_channel4" ("mux10_1(x6)_encode")) -> (Variant=w12119:variant)
                n5540 = To Variant(anything=T4."demux1_10_channel4" ("demux1_10(x6)_encode")) -> (Variant=w12115:variant)
                n5541 = To Variant(anything=bool[] [FALSE, FALSE, FALSE, FALSE, TRUE, FALSE]) -> (Variant=w12130:variant)
                n5542 = Bundle By Name(cluster=w12121, "command"="MEAS.AllRelaysOFF") -> (w12129:T9)
                n5543 = Bundle By Name(cluster=w12121, "command"="MEAS.mux10-1", "data"=w12119) -> (w12112:T9)
                n5544 = Bundle By Name(cluster=w12121, "command"="MEAS.demux1-10", "data"=w12115) -> (w12113:T9)
                n5545 = Bundle By Name(cluster=w12121, "command"="MEAS.eMIC", "data"=w12130) -> (w12114:T9)
                n5546 = Build Array(w12129, w12112, w12113, w12114) -> (w12107:T9[])
                n5547 = To Variant(anything=w12111) -> (Variant=w12110:variant)
                n5548 = To Variant(anything=w12111) -> (Variant=w12109:variant)
                n5549 = Bundle By Name(cluster=w12108, "command"="MEAS.requestAC", "data"=w12110) -> (w12127:T9)
                n5550 = Bundle By Name(cluster=w12108, "command"="Apps.WaitForEvent", "data"=w12109) -> (w12123:T9)
                n5551 = Bundle By Name(cluster=w12108, "command"="Apps.UI Update 1") -> (w12124:T9)
                n5552 = Bundle By Name(cluster=w12108, "command"="WaitFor") -> (w12106:T9)
                n5553 = Build Array (concatenate)(w12107, w12106, w12127, w12123, w12124) -> (w12122:T9[])
              }
              frame True {
                w12137 = T9 {"command"="", "data"=variant} ("element")
                w12159 = T9 {"command"="", "data"=variant} ("element")
                n5554 = To Variant(anything=T3."mux10_1_channel4" ("mux10_1(x6)_encode")) -> (Variant=w12166:variant)
                n5555 = To Variant(anything=T2."mux6_1_channel5_3" ("mux6_1(3wires)_encode")) -> (Variant=w12164:variant)
                n5556 = To Variant(anything=T4."demux1_10_channel4" ("demux1_10(x6)_encode")) -> (Variant=w12160:variant)
                n5557 = To Variant(anything=bool[] [FALSE, FALSE, FALSE, FALSE, TRUE, FALSE]) -> (Variant=w12156:variant)
                n5558 = Bundle By Name(cluster=w12159, "command"="MEAS.AllRelaysOFF") -> (w12155:T9)
                n5559 = Bundle By Name(cluster=w12159, "command"="MEAS.mux10-1", "data"=w12166) -> (w12154:T9)
                n5560 = Bundle By Name(cluster=w12159, "command"="MEAS.mux6_1", "data"=w12164) -> (w12153:T9)
                n5561 = Bundle By Name(cluster=w12159, "command"="MEAS.demux1-10", "data"=w12160) -> (w12152:T9)
                n5562 = Bundle By Name(cluster=w12159, "command"="MEAS.eMIC", "data"=w12156) -> (w12151:T9)
                n5563 = Build Array(w12155, w12154, w12153, w12152, w12151) -> (w12136:T9[])
                n5564 = To Variant(anything=w12141) -> (Variant=w12139:variant)
                n5565 = To Variant(anything=w12141) -> (Variant=w12138:variant)
                n5566 = Bundle By Name(cluster=w12137, "command"="WaitFor") -> (w12135:T9)
                n5567 = Bundle By Name(cluster=w12137, "command"="MEAS.DMM dual read") -> (w12148:T9)
                n5568 = Bundle By Name(cluster=w12137, "command"="MEAS.requestAC", "data"=w12139) -> (w12147:T9)
                n5569 = Bundle By Name(cluster=w12137, "command"="Apps.WaitForEvent", "data"=w12138) -> (w12142:T9)
                n5570 = Bundle By Name(cluster=w12137, "command"="Apps.UI Update 1") -> (w12143:T9)
                n5571 = Build Array (concatenate)(w12136, w12135, w12148, w12147, w12142, w12143) -> (w12140:T9[])
              }
            }
          }
          frame True {
            n5572 = Bundle By Name(cluster=T9 {"command"="", "data"=variant} ("element"), "command"="Apps.UI Update 1") -> (w12170:T9)
            n5573 = Build Array(w12170) -> (w12169:T9[])
          }
        }
        n5574 = for {
          tunnel: w12085 -> [w12180] mode=indexing
          tunnel: w12093 -> [w12181]
          tunnel: [w12177] -> w12095 mode=indexing
          n5575 = Unbundle By Name(w12180) -> ("command"=w12179:string, "data"=w12178:variant)
          n5576 = call "App enquece.vi"("command data"=w12178, "command"=w12179, "queue in"=w12181) -> ("error out"=w12177:errorcluster)  [unwired: 7 in, 1 out]
        }
        n5577 = Merge Errors(w12096, w12095) -> (w12094:errorcluster)
      }
      frame "Test DRV 24A" {
        w12185 = 24 ("DUT index(0-59)")
        n5578 = disable-structure shown="LOGGING==TRUE" {
          disable-tunnel: w12190 -> [w12273 _]
          frame condition #0 (active) {
            n5579 = Empty String/Path?(string/path=w12273) -> (empty?=w12275:bool)
            n5580 = Select(t="Quece timeout", s=w12275, f=w12273) -> (s? t:f=w12272:string)
            n5581 = call "string log (SubVI).vi"("state Name"=w12272) -> ()  [unwired: 9 in, 2 out]
          }
          frame condition #1 {
          }
        }
        n5582 = Flush Queue(queue=w12191) -> (queue out=w12192:refnum<queue>)  [unwired: 1 in, 2 out]
        n5583 = Decrement(x=w12185) -> (x-1=w12189:i32)
        n5584 = Index Array(array=w12186, index=w12189) -> (element=w12187:refnum<vi>)
        n5585 = call "FGV DRV stand.vi"() -> ("Sub-Test.DCV"=w12182:bool)  [unwired: 10 in, 1 out]
        n5586 = call "FGV Driver Data.vi"("DUT index(1-60)"=w12185) -> ("DUT SC"=w12183:bool)  [unwired: 7 in, 3 out]
        n5587 = property class="ColBox"(reference=w12187, "Value"=u32 10000536 ("DRV 1")) -> ()  [unwired: 1 in, 2 out]
        n5588 = case shown="False" w12183 {
          tunnel: w12185 -> [w12203 _]
          tunnel: [w12202 w12268] -> w12184
          tunnel: w12182 -> [w12201 _]
          frame False {
            n5589 = case shown="False" w12201 {
              tunnel: w12203 -> [w12210 w12240]
              tunnel: [w12221 w12239] -> w12202
              frame False {
                w12207 = T9 {"command"="", "data"=variant} ("element")
                w12220 = T9 {"command"="", "data"=variant} ("element")
                n5590 = To Variant(anything=T3."mux10_1_channel4" ("mux10_1(x6)_encode")) -> (Variant=w12218:variant)
                n5591 = To Variant(anything=T4."demux1_10_channel4" ("demux1_10(x6)_encode")) -> (Variant=w12214:variant)
                n5592 = To Variant(anything=bool[] [FALSE, FALSE, FALSE, FALSE, FALSE, TRUE]) -> (Variant=w12229:variant)
                n5593 = Bundle By Name(cluster=w12220, "command"="MEAS.AllRelaysOFF") -> (w12228:T9)
                n5594 = Bundle By Name(cluster=w12220, "command"="MEAS.mux10-1", "data"=w12218) -> (w12211:T9)
                n5595 = Bundle By Name(cluster=w12220, "command"="MEAS.demux1-10", "data"=w12214) -> (w12212:T9)
                n5596 = Bundle By Name(cluster=w12220, "command"="MEAS.eMIC", "data"=w12229) -> (w12213:T9)
                n5597 = Build Array(w12228, w12211, w12212, w12213) -> (w12206:T9[])
                n5598 = To Variant(anything=w12210) -> (Variant=w12209:variant)
                n5599 = To Variant(anything=w12210) -> (Variant=w12208:variant)
                n5600 = Bundle By Name(cluster=w12207, "command"="MEAS.requestAC", "data"=w12209) -> (w12226:T9)
                n5601 = Bundle By Name(cluster=w12207, "command"="Apps.WaitForEvent", "data"=w12208) -> (w12222:T9)
                n5602 = Bundle By Name(cluster=w12207, "command"="Apps.UI Update 1") -> (w12223:T9)
                n5603 = Bundle By Name(cluster=w12207, "command"="WaitFor") -> (w12205:T9)
                n5604 = Build Array (concatenate)(w12206, w12205, w12226, w12222, w12223) -> (w12221:T9[])
              }
              frame True {
                w12236 = T9 {"command"="", "data"=variant} ("element")
                w12258 = T9 {"command"="", "data"=variant} ("element")
                n5605 = To Variant(anything=T3."mux10_1_channel4" ("mux10_1(x6)_encode")) -> (Variant=w12265:variant)
                n5606 = To Variant(anything=T2."mux6_1_channel6_3" ("mux6_1(3wires)_encode")) -> (Variant=w12263:variant)
                n5607 = To Variant(anything=T4."demux1_10_channel4" ("demux1_10(x6)_encode")) -> (Variant=w12259:variant)
                n5608 = To Variant(anything=bool[] [FALSE, FALSE, FALSE, FALSE, FALSE, TRUE]) -> (Variant=w12255:variant)
                n5609 = Bundle By Name(cluster=w12258, "command"="MEAS.AllRelaysOFF") -> (w12254:T9)
                n5610 = Bundle By Name(cluster=w12258, "command"="MEAS.mux10-1", "data"=w12265) -> (w12253:T9)
                n5611 = Bundle By Name(cluster=w12258, "command"="MEAS.mux6_1", "data"=w12263) -> (w12252:T9)
                n5612 = Bundle By Name(cluster=w12258, "command"="MEAS.demux1-10", "data"=w12259) -> (w12251:T9)
                n5613 = Bundle By Name(cluster=w12258, "command"="MEAS.eMIC", "data"=w12255) -> (w12250:T9)
                n5614 = Build Array(w12254, w12253, w12252, w12251, w12250) -> (w12235:T9[])
                n5615 = To Variant(anything=w12240) -> (Variant=w12238:variant)
                n5616 = To Variant(anything=w12240) -> (Variant=w12237:variant)
                n5617 = Bundle By Name(cluster=w12236, "command"="WaitFor") -> (w12234:T9)
                n5618 = Bundle By Name(cluster=w12236, "command"="MEAS.DMM dual read") -> (w12247:T9)
                n5619 = Bundle By Name(cluster=w12236, "command"="MEAS.requestAC", "data"=w12238) -> (w12246:T9)
                n5620 = Bundle By Name(cluster=w12236, "command"="Apps.WaitForEvent", "data"=w12237) -> (w12241:T9)
                n5621 = Bundle By Name(cluster=w12236, "command"="Apps.UI Update 1") -> (w12242:T9)
                n5622 = Build Array (concatenate)(w12235, w12234, w12247, w12246, w12241, w12242) -> (w12239:T9[])
              }
            }
          }
          frame True {
            n5623 = Bundle By Name(cluster=T9 {"command"="", "data"=variant} ("element"), "command"="Apps.UI Update 1") -> (w12269:T9)
            n5624 = Build Array(w12269) -> (w12268:T9[])
          }
        }
        n5625 = for {
          tunnel: w12184 -> [w12279] mode=indexing
          tunnel: w12192 -> [w12280]
          tunnel: [w12276] -> w12194 mode=indexing
          n5626 = Unbundle By Name(w12279) -> ("command"=w12278:string, "data"=w12277:variant)
          n5627 = call "App enquece.vi"("command data"=w12277, "command"=w12278, "queue in"=w12280) -> ("error out"=w12276:errorcluster)  [unwired: 7 in, 1 out]
        }
        n5628 = Merge Errors(w12195, w12194) -> (w12193:errorcluster)
      }
      frame "Test DRV 25A" {
        w12284 = 25 ("DUT index(0-59)")
        n5629 = disable-structure shown="LOGGING==TRUE" {
          disable-tunnel: w12289 -> [w12372 _]
          frame condition #0 (active) {
            n5630 = Empty String/Path?(string/path=w12372) -> (empty?=w12374:bool)
            n5631 = Select(t="Quece timeout", s=w12374, f=w12372) -> (s? t:f=w12371:string)
            n5632 = call "string log (SubVI).vi"("state Name"=w12371) -> ()  [unwired: 9 in, 2 out]
          }
          frame condition #1 {
          }
        }
        n5633 = Flush Queue(queue=w12290) -> (queue out=w12291:refnum<queue>)  [unwired: 1 in, 2 out]
        n5634 = Decrement(x=w12284) -> (x-1=w12288:i32)
        n5635 = Index Array(array=w12285, index=w12288) -> (element=w12286:refnum<vi>)
        n5636 = call "FGV DRV stand.vi"() -> ("Sub-Test.DCV"=w12281:bool)  [unwired: 10 in, 1 out]
        n5637 = call "FGV Driver Data.vi"("DUT index(1-60)"=w12284) -> ("DUT SC"=w12282:bool)  [unwired: 7 in, 3 out]
        n5638 = property class="ColBox"(reference=w12286, "Value"=u32 10000536 ("DRV 1")) -> ()  [unwired: 1 in, 2 out]
        n5639 = case shown="False" w12282 {
          tunnel: w12284 -> [w12302 _]
          tunnel: [w12301 w12367] -> w12283
          tunnel: w12281 -> [w12300 _]
          frame False {
            n5640 = case shown="True" w12300 {
              tunnel: w12302 -> [w12309 w12339]
              tunnel: [w12320 w12338] -> w12301
              frame False {
                w12306 = T9 {"command"="", "data"=variant} ("element")
                w12319 = T9 {"command"="", "data"=variant} ("element")
                n5641 = To Variant(anything=T3."mux10_1_channel5" ("mux10_1(x6)_encode")) -> (Variant=w12317:variant)
                n5642 = To Variant(anything=T4."demux1_10_channel5" ("demux1_10(x6)_encode")) -> (Variant=w12313:variant)
                n5643 = To Variant(anything=bool[] [TRUE, FALSE, FALSE, FALSE, FALSE, FALSE]) -> (Variant=w12328:variant)
                n5644 = Bundle By Name(cluster=w12319, "command"="MEAS.AllRelaysOFF") -> (w12327:T9)
                n5645 = Bundle By Name(cluster=w12319, "command"="MEAS.mux10-1", "data"=w12317) -> (w12310:T9)
                n5646 = Bundle By Name(cluster=w12319, "command"="MEAS.demux1-10", "data"=w12313) -> (w12311:T9)
                n5647 = Bundle By Name(cluster=w12319, "command"="MEAS.eMIC", "data"=w12328) -> (w12312:T9)
                n5648 = Build Array(w12327, w12310, w12311, w12312) -> (w12305:T9[])
                n5649 = To Variant(anything=w12309) -> (Variant=w12308:variant)
                n5650 = To Variant(anything=w12309) -> (Variant=w12307:variant)
                n5651 = Bundle By Name(cluster=w12306, "command"="MEAS.requestAC", "data"=w12308) -> (w12325:T9)
                n5652 = Bundle By Name(cluster=w12306, "command"="Apps.WaitForEvent", "data"=w12307) -> (w12321:T9)
                n5653 = Bundle By Name(cluster=w12306, "command"="Apps.UI Update 1") -> (w12322:T9)
                n5654 = Bundle By Name(cluster=w12306, "command"="WaitFor") -> (w12304:T9)
                n5655 = Build Array (concatenate)(w12305, w12304, w12325, w12321, w12322) -> (w12320:T9[])
              }
              frame True {
                w12335 = T9 {"command"="", "data"=variant} ("element")
                w12357 = T9 {"command"="", "data"=variant} ("element")
                n5656 = To Variant(anything=T3."mux10_1_channel5" ("mux10_1(x6)_encode")) -> (Variant=w12364:variant)
                n5657 = To Variant(anything=T2."mux6_1_channel1_3" ("mux6_1(3wires)_encode")) -> (Variant=w12362:variant)
